vi "encoders.vi"   [LabVIEW 2012]
uses:
  Robot Global Data.vi
types:
  T1 = typedef "WPI_EncoderDevRef.ctl" = cluster{"DevStatus":errorcluster, "EncoderIndex":T2, "CounterIndex":T3, "DistancePerCount":dbl, "Decoding Type":T4}
  T2 = typedef "FPGA_EncoderIdx.ctl" = enum8{"Enc 0", "Enc 1", "Enc 2", "Enc 3", "Invalid"}
  T3 = typedef "FPGA_CounterCtrSystemIndex.ctl" = enum8{"Ctr 0", "Ctr 1", "Ctr 2", "Ctr 3", "Ctr 4", "Ctr 5", "Ctr 6", "Ctr 7", "Invalid"}
  T4 = typedef "WPI_EncoderType.ctl" = enum16{"1x", "2x", "4x"}
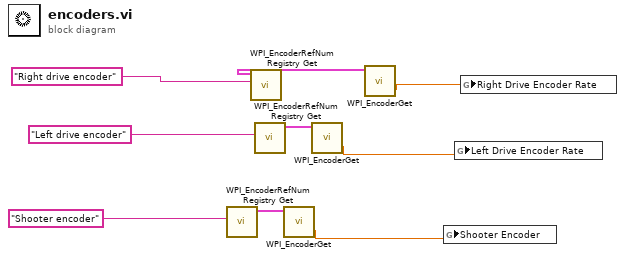
[diagram p0: block diagram]
diagram:
  n1 = call <vilib>:"WPI_EncoderRefNum Registry Get.vi"("refnum name"="Shooter encoder") -> ("EncoderDevRef"=w2:T1)  [unwired: 9 in, 1 out]
  n2 = call <vilib>:"WPI_EncoderRefNum Registry Get.vi"("refnum name"="Right drive encoder") -> ("EncoderDevRef"=w8:T1)  [unwired: 9 in, 1 out]
  n3 = call <vilib>:"WPI_EncoderRefNum Registry Get.vi"("refnum name"="Left drive encoder") -> ("EncoderDevRef"=w6:T1)  [unwired: 9 in, 1 out]
  n4 = call <vilib>:"WPI_EncoderGet.vi"("EncoderDevRef"=w2) -> ("Rate"=w1:dbl)  [unwired: 5 in, 5 out]
  n5 = call <vilib>:"WPI_EncoderGet.vi"("EncoderDevRef"=w6) -> ("Rate"=w4:dbl)  [unwired: 5 in, 5 out]
  n6 = call <vilib>:"WPI_EncoderGet.vi"("EncoderDevRef"=w8) -> ("Rate"=w5:dbl)  [unwired: 5 in, 5 out]
  n7 = global write "Robot Global Data.vi" "Shooter Encoder"(w1) -> ()
  n8 = global write "Robot Global Data.vi" "Left Drive Encoder Rate"(w4) -> ()
  n9 = global write "Robot Global Data.vi" "Right Drive Encoder Rate"(w5) -> ()
